vi "ODMR sweep ACCES DAC control low freq.vi"(8 "Save?":bool, 9 "file path (dialog if empty)":path=path "C:/Users/Ouyang Group/Documents/Data/8-12-16/MNP 2 new on CPW 2mW scan 2 x35 y103 ODMR B0.5V T90 rf", 10 "Cluster":T1={"Freq start"=50000000.0, "Freq End"=1000000000.0, "Freq Step"=5000000.0, "Power (dbm)"=-4.0, "number of samples per channel"=200}, 11 "Dot Tracking Cluster":T3={"RS232 settings"={"Portnumber"=12, "Baudrate"=5}, "X Parameters"={"Number of X Steps"=200, "Max X (V)"=2.0, "Min X (V)"=-2.0}, "Y Parameters"={"Number of Y Steps"=200, "Max Y (V)"=2.0, "Min Y (V)"=-2.0}, "X Pos"=75.0, "Y Pos"=145.0, "Z Pos"=52.78, "Tracking interval"=150.0} {"RS232 settings"."Portnumber" items=["COM1", "COM2", "COM3", "COM4", "COM5", "COM6", "COM7", "COM8", "COM9", "COM10", "COM11", "COM12", "COM13", "COM14", "COM15", "COM16", "COM17", "COM18", "COM19", "COM20", "COM21", "COM22", "COM23", "COM24", "COM25", "COM26", "COM27", "COM28", "COM29", "COM30"]; "RS232 settings"."Baudrate" items=["9600", "14400", "19200", "38400", "57600", "115200"]}) -> (0 "Z Position":dbl=31.0, 1 "Y Position":dbl=62.0, 2 "X Position":dbl=97.0, 3 "XY Graph":cluster{"Y":dbl[], "Y":dbl[]}[](graph), 4 "appended array":ext[][](array[numeric]))   [LabVIEW 2012]
uses:
  <vilib>/DAQmx/read.llb/DAQmx Read (Counter 1D DBL 1Chan NSamp).vi
  <vilib>/DAQmx/create/channels.llb/DAQmx Create Channel (CI-Count Edges).vi
  <vilib>/DAQmx/configure/timing.llb/DAQmx Timing (Sample Clock).vi
  <vilib>/Instr/_visa.llb/VISA Configure Serial Port (Instr).vi
  <vilib>/DAQmx/miscellaneous.llb/DAQmx Fill In Error Info.vi
  <vilib>/Utility/file.llb/Write To Spreadsheet File (DBL).vi
  <resource>/objmgr/daqmx.rc
panel:
  in  "Serial Cluster":T2={"baud rate"=4800, "VISA resource name"="COM8", "data bits"=8, "parity"=0, "stop bits"=10, "flow control"=0} {"flow control" items=["None"=0, "XON/XOFF"=1, "RTS/CTS"=2, "DTR/DSR"=4]; "stop bits" items=["1.0"=10, "1.5"=15, "2.0"=20]; "parity" items=["None", "Odd", "Even", "Mark", "Space"]; "data bits" min=5 max=8 step=1}
  in  "stop":bool
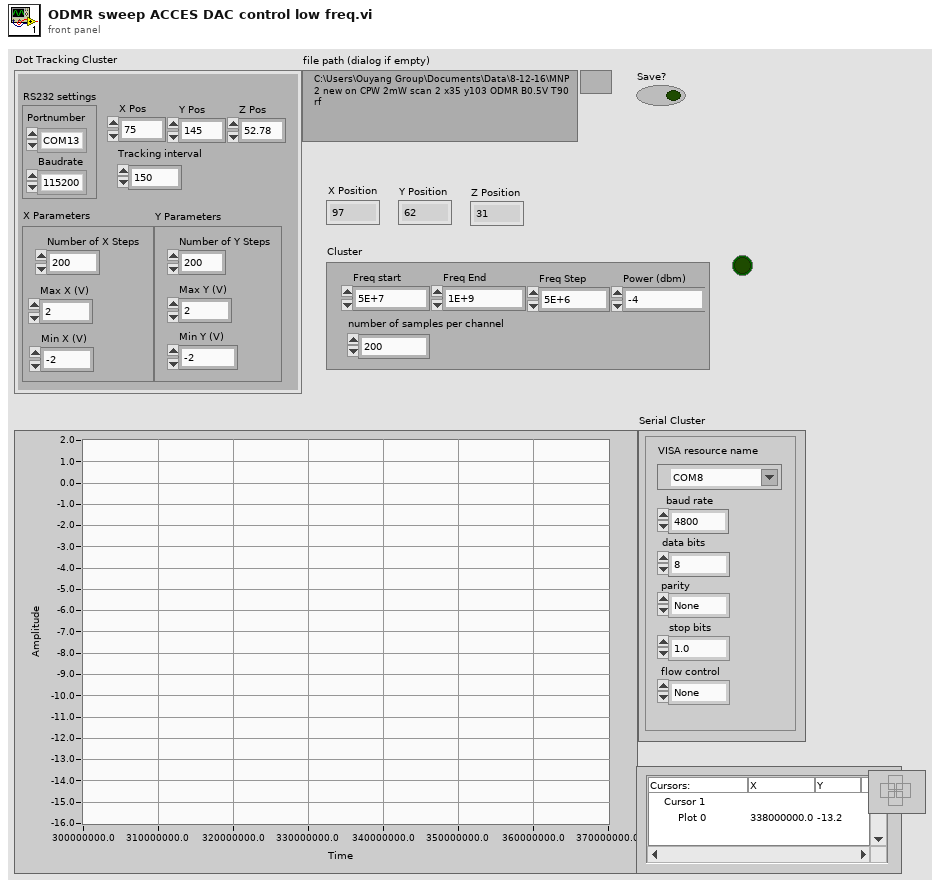
[diagram p1: front panel]
types:
  T1 = cluster{"Freq start":dbl, "Freq End":dbl, "Freq Step":dbl, "Power (dbm)":dbl, "number of samples per channel":i32}
  T2 = cluster{"baud rate":u32, "VISA resource name":refnum<visa-resource-name>, "data bits":u16, "parity":u16, "stop bits":u16, "flow control":u16}
  T3 = cluster{"RS232 settings":cluster{"Portnumber":i32, "Baudrate":u16}, "X Parameters":cluster{"Number of X Steps":i32, "Max X (V)":dbl, "Min X (V)":dbl}, "Y Parameters":cluster{"Number of Y Steps":i32, "Max Y (V)":dbl, "Min Y (V)":dbl}, "X Pos":dbl, "Y Pos":dbl, "Z Pos":dbl, "Tracking interval":dbl}
  T4 = cluster{"Number of X Steps":i32, "Max X (V)":dbl, "Min X (V)":dbl}
  T5 = cluster{"Number of Y Steps":i32, "Max Y (V)":dbl, "Min Y (V)":dbl}
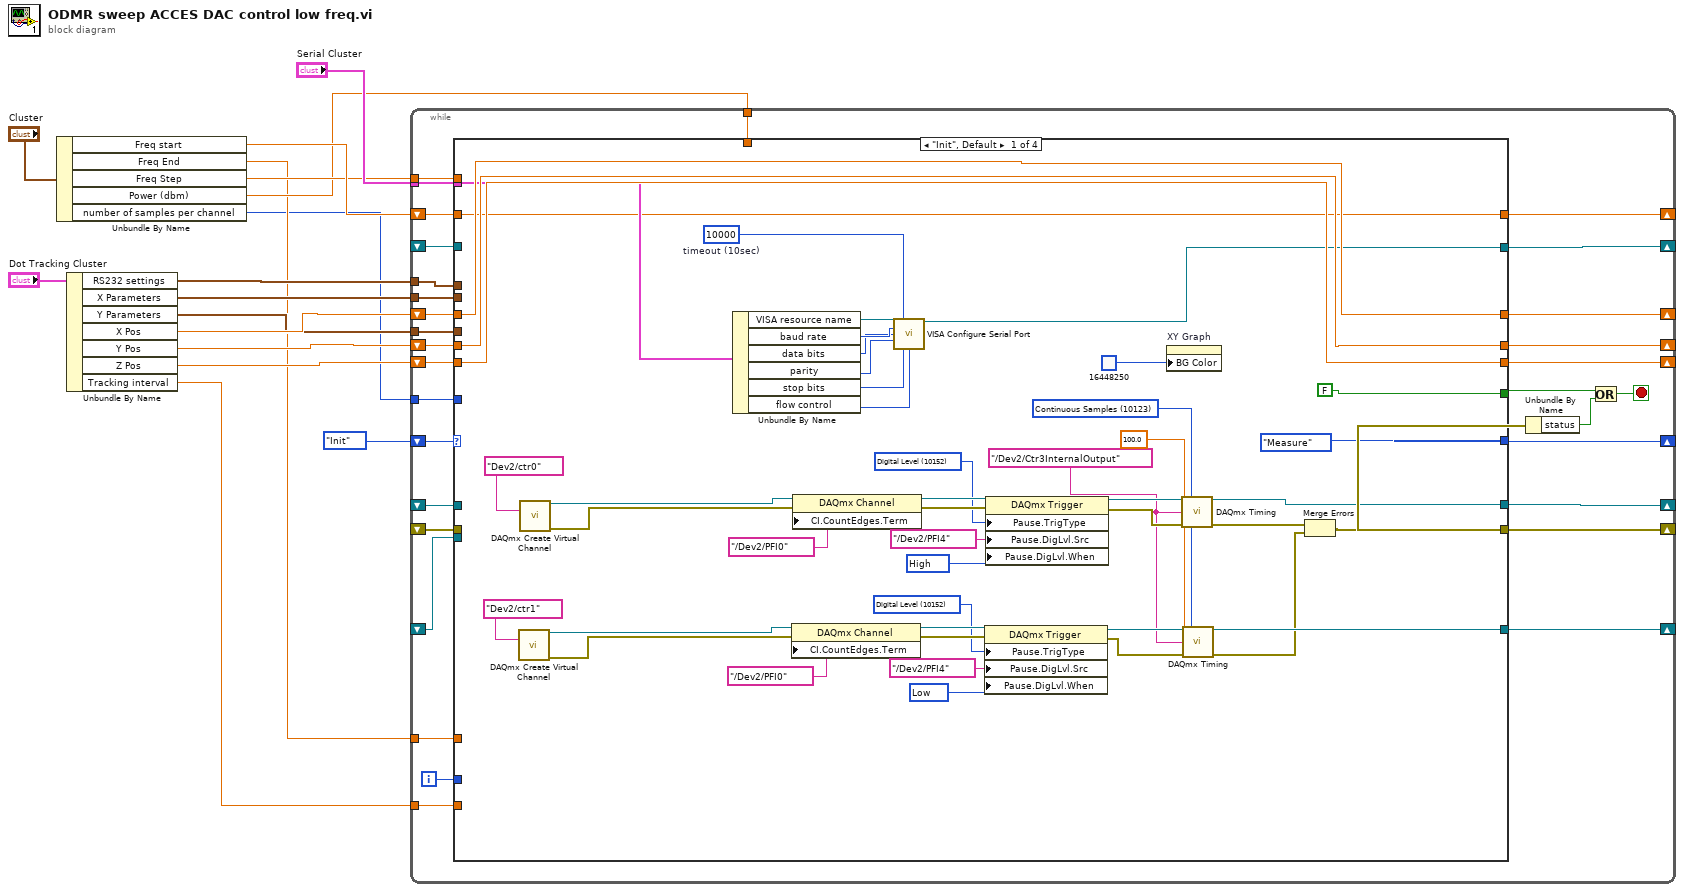
[diagram p0: block diagram]
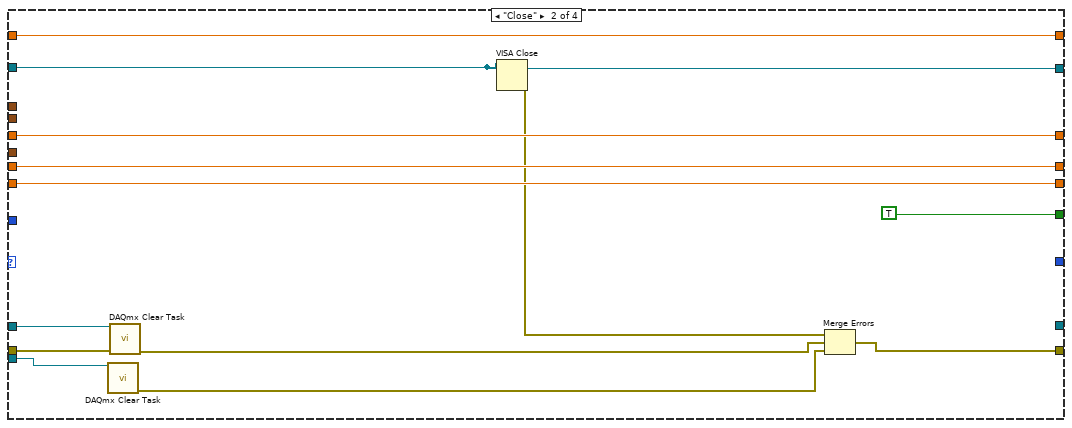
[diagram p2: hidden frame]
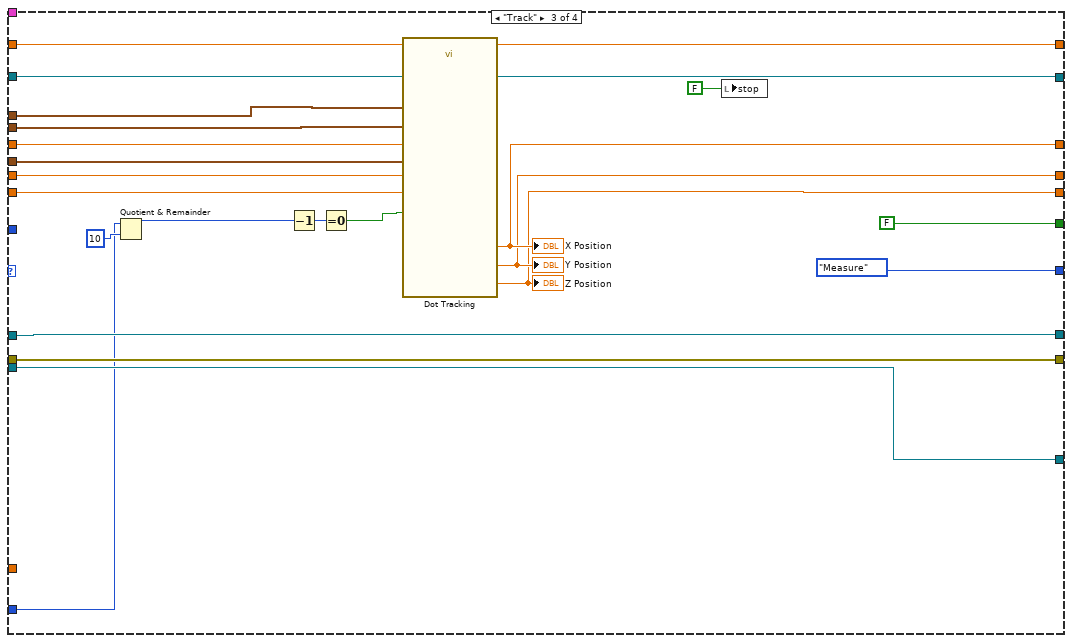
[diagram p3: hidden frame]
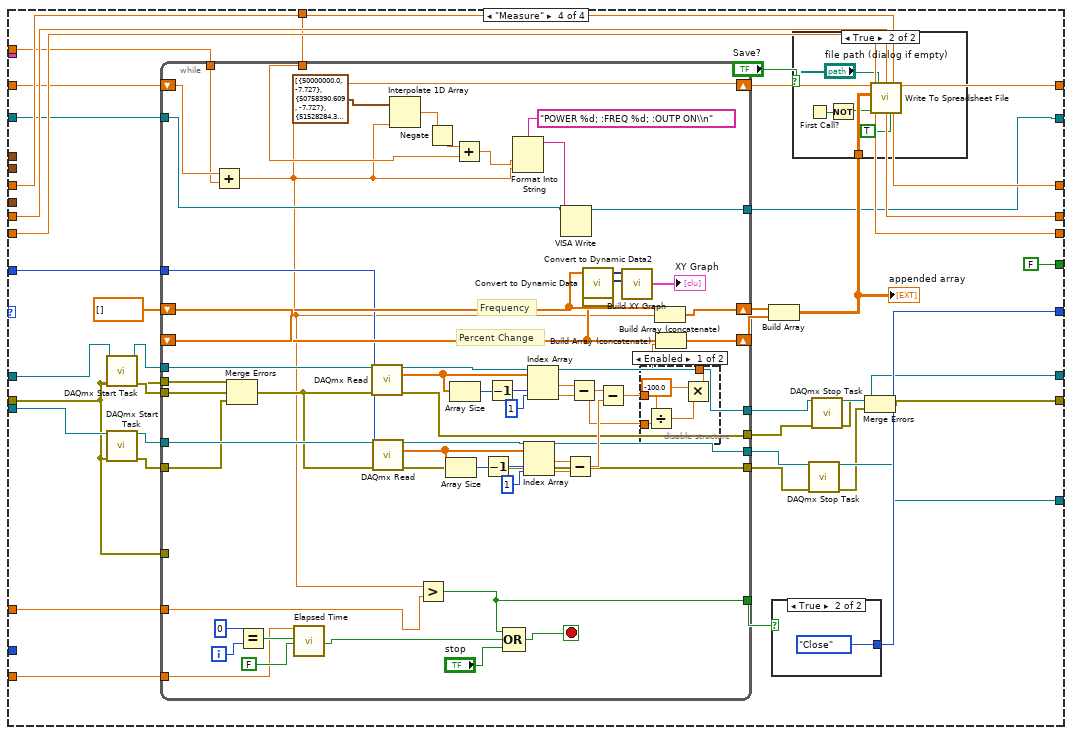
[diagram p4: hidden frame]
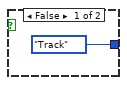
[diagram p6: hidden frame]
diagram:
  n1 = Unbundle By Name("Cluster") -> ("Freq start"=w5:dbl, "Freq End"=w2:dbl, "Freq Step"=w4:dbl, "Power (dbm)"=w3:dbl, "number of samples per channel"=w1:i32)
  n2 = Unbundle By Name("Dot Tracking Cluster") -> ("RS232 settings"=w11:cluster{"Portnumber":i32, "Baudrate":u16}, "X Parameters"=w10:T4, "Y Parameters"=w9:T5, "X Pos"=w14:dbl, "Y Pos"=w13:dbl, "Z Pos"=w12:dbl, "Tracking interval"=w8:dbl)
  n3 = while {
    shift-right: [w44] -> _
    shift-left: enum16{"Init", "Measure", "Track", "Close"}."Init" -> [w47]
    shift-right: [w46] -> _
    shift-left: _ -> [w43]
    shift-right: [w45] -> _
    shift-left: _ -> [w42]
    shift-right: [w40] -> _
    shift-left: _ -> [w41]
    shift-right: [w33] -> _
    shift-left: w14 -> [w36]
    shift-right: [w32] -> _
    shift-left: w13 -> [w35]
    shift-right: [w31] -> _
    shift-left: w12 -> [w34]
    tunnel: w11 -> [w30]
    tunnel: w10 -> [w29]
    tunnel: w9 -> [w28]
    tunnel: w8 -> [w27]
    tunnel: "Serial Cluster" -> [w26]
    tunnel: w3 -> [w25]
    shift-right: [w21] -> _
    shift-left: w5 -> [w24]
    shift-right: [w23] -> _
    shift-left: _ -> [w22]
    tunnel: w4 -> [w20]
    tunnel: w2 -> [w19]
    tunnel: w1 -> [w18]
    i -> [w17]
    stop <- w39 stop-if-true
    n4 = case shown="\"Init\", Default" w47 {
      tunnel: [FALSE TRUE FALSE FALSE] -> w38
      tunnel: [w69 _ w128 w154] -> w46
      tunnel: [w68 _ w127 w151] -> w45
      tunnel: [w65 w101 w122 w164] -> w40
      tunnel: [enum16{"Init", "Measure", "Track", "Close"}."Measure" _ enum16{"Init", "Measure", "Track", "Close"}."Measure" w163] -> w44
      tunnel: w43 -> [_ w105 w128 w160]
      tunnel: w42 -> [_ w103 w127 w157]
      tunnel: w41 -> [_ w104 w122 w141]
      tunnel: w36 -> [w61 w99 w118 w146]
      tunnel: w35 -> [w60 w98 w117 w145]
      tunnel: w34 -> [w59 w97 w116 w144]
      tunnel: [w61 w99 w115 w146] -> w33
      tunnel: [w60 w98 w114 w145] -> w32
      tunnel: [w59 w97 w113 w144] -> w31
      tunnel: w30 -> [_ _ w112 _]
      tunnel: w29 -> [_ _ w111 _]
      tunnel: w28 -> [_ _ w110 _]
      tunnel: w27 -> [_ _ _ w140]
      tunnel: w26 -> [w51 _ _ _]
      tunnel: w25 -> [_ _ _ w136]
      tunnel: w24 -> [w49 w94 w108 w135]
      tunnel: [w50 w95 w109 w133] -> w23
      tunnel: w22 -> [_ w95 w109 w134]
      tunnel: [w49 w94 w108 w132] -> w21
      tunnel: w20 -> [_ _ _ w131]
      tunnel: w19 -> [_ _ _ w130]
      tunnel: w18 -> [_ _ _ w129]
      tunnel: w17 -> [_ _ w107 _]
      frame "Init", Default {
        w48 = 100.0 ("rate")
        w58 = u32 10000  # timeout (10sec)
        w70 = tag "/Dev2/Ctr3InternalOutput" ("source")
        w71 = 10123 items=["Finite Samples"=10178, "Continuous Samples"=10123, "Hardware Timed Single Point"=12522] ("sample mode")
        w76 = 10214 items=["High"=10192, "Low"=10214] ("Pause.DigLvl.When")
        w78 = 10152 items=["Analog Level"=10101, "Analog Window"=10103, "Digital Level"=10152, "Digital Pattern"=10398, "None"=10230] ("Pause.TrigType")
        w85 = 10192 items=["High"=10192, "Low"=10214] ("Pause.DigLvl.When")
        w87 = 10152 items=["Analog Level"=10101, "Analog Window"=10103, "Digital Level"=10152, "Digital Pattern"=10398, "None"=10230] ("Pause.TrigType")
        n5 = call-poly <vilib>:"DAQmx Create Virtual Channel.vi"("counter"=tag "Dev2/ctr1") -> ("task out"=w83:refnum<k21>, "error out"=w82:errorcluster)  [unwired: 13 in]
        n6 = call-poly <vilib>:"DAQmx Create Virtual Channel.vi"("counter"=tag "Dev2/ctr0") -> ("task out"=w92:refnum<k21>, "error out"=w91:errorcluster)  [unwired: 13 in]
        n7 = Unbundle By Name(w51) -> ("VISA resource name"=w57:refnum<visa-resource-name>, "baud rate"=w56:u32, "data bits"=w55:u16, "parity"=w54:u16, "stop bits"=w53:u16, "flow control"=w52:u16)
        n8 = property class="DAQmx Channel"(reference=w83, error in=w82, "CI.CountEdges.Term"=tag "/Dev2/PFI0") -> (reference out=w80:refnum<k21>, error out=w79:errorcluster)
        n9 = property class="DAQmx Channel"(reference=w92, error in=w91, "CI.CountEdges.Term"=tag "/Dev2/PFI0") -> (reference out=w89:refnum<k21>, error out=w88:errorcluster)
        n10 = call-poly "VISA Configure Serial Port"("VISA resource name"=w57, "timeout (10sec)"=w58, "baud rate (9600)"=w56, "data bits (8)"=w55, "parity (0:none)"=w54, "stop bits (10: 1 bit)"=w53, "flow control (0:none)"=w52) -> ("VISA resource name out"=w50:refnum<visa-resource-name>)  [unwired: 2 in, 6 out]
        n11 = property class="DAQmx Trigger"(reference=w80, error in=w79, "Pause.TrigType"=w78, "Pause.DigLvl.Src"=tag "/Dev2/PFI4", "Pause.DigLvl.When"=w76) -> (reference out=w73:refnum<k21>, error out=w72:errorcluster)
        n12 = property class="DAQmx Trigger"(reference=w89, error in=w88, "Pause.TrigType"=w87, "Pause.DigLvl.Src"=tag "/Dev2/PFI4", "Pause.DigLvl.When"=w85) -> (reference out=w75:refnum<k21>, error out=w74:errorcluster)
        n13 = property on="XY Graph" class="XYGraph (strict)"("BG Color"=u32 16448250) -> ()  [unwired: 2 in, 2 out]
        n14 = call-poly <vilib>:"DAQmx Timing.vi"("task/channels in"=w75, "sample mode"=w71, "rate"=w48, "source"=w70, "error in"=w74) -> ("task out"=w69:refnum<k21>, "error out"=w67:errorcluster)  [unwired: 9 in]
        n15 = call-poly <vilib>:"DAQmx Timing.vi"("task/channels in"=w73, "sample mode"=w71, "rate"=w48, "source"=w70, "error in"=w72) -> ("task out"=w68:refnum<k21>, "error out"=w66:errorcluster)  [unwired: 9 in]
        n16 = Merge Errors(w67, w66) -> (w65:errorcluster)
      }
      frame "Close" {
        n17 = call <vilib>:"DAQmx Clear Task.vi"("task in"=w103) -> ("error out"=w102:errorcluster)  [unwired: 14 in]
        n18 = call <vilib>:"DAQmx Clear Task.vi"("task in"=w105, "error in"=w104) -> ("error out"=w100:errorcluster)  [unwired: 13 in]
        n19 = VISA Close(VISA resource name=w95) -> (error out=w96:errorcluster)  [unwired: 1 in]
        n20 = Merge Errors(w96, w100, w102) -> (w101:errorcluster)
      }
      frame "Track" {
        n21 = Quotient & Remainder(x=w107, y=10) -> (x-y*floor(x/y)=w125:i32)  [unwired: 1 out]
        n22 = Decrement(x=w125) -> (x-1=w126:i32)
        n23 = Equal To 0?(x=w126) -> (x = 0?=w123:bool)
        n24 = call "Dot Tracking.vi"("X"=w111, "Y Parameters"=w110, "RS232 settings"=w112, "X Pos"=w118, "Y pos"=w117, "Z Pos"=w116, "Z-track?"=w123) -> ("X Position"=w115:dbl, "Y Position"=w114:dbl, "Z Position"=w113:dbl)  [unwired: 2 in, 4 out]
        "X Position" <- w115
        "Y Position" <- w114
        "Z Position" <- w113
        n25 = local write "stop"(FALSE ("stop")) -> ()
      }
      frame "Measure" {
        w147 = dbl[] []
        n26 = call <vilib>:"DAQmx Start Task.vi"("task/channels in"=w160, "error in"=w141) -> ("task out"=w158:refnum<k21>, "error out"=w159:errorcluster)  [unwired: 12 in]
        n27 = call <vilib>:"DAQmx Start Task.vi"("task/channels in"=w157, "error in"=w141) -> ("task out"=w156:refnum<k21>, "error out"=w155:errorcluster)  [unwired: 12 in]
        n28 = while {
          shift-right: [w214] -> w149
          shift-left: w147 -> [w202]
          shift-right: [w213] -> w139
          shift-left: w147 -> [w204]
          tunnel: w156 -> [w210]
          tunnel: [w209] -> w153
          tunnel: [w208] -> w162
          tunnel: [w205] -> w161
          tunnel: w159 -> [w207]
          tunnel: w158 -> [w206]
          tunnel: w155 -> [w191]
          tunnel: w141 -> [w186]
          tunnel: [w189] -> w143
          tunnel: [w188] -> w142
          tunnel: w141 -> [_]
          tunnel: w140 -> [w187]
          tunnel: w136 -> [w174]
          shift-right: [w172] -> w132
          shift-left: w135 -> [w183]
          tunnel: w134 -> [w182]
          tunnel: [w181] -> w133
          tunnel: w131 -> [w180]
          tunnel: w130 -> [w179]
          tunnel: w129 -> [w178]
          i -> [w196]
          stop <- w192 stop-if-true
          # "Percent Change"
          # "Frequency"
          n29 = Add(x=w183, y=w180) -> (x+y=w172:dbl)
          n30 = Merge Errors(w186, w207, w191) -> (w190:errorcluster)
          n31 = Equal?(x=0, y=w196) -> (x = y?=w195:bool)
          n32 = call "Elapsed Time"("Time Target (s)"=w187, "Reset"=w195, "Auto Reset"=FALSE) -> ("Time has Elapsed"=w194:bool)  [unwired: 9 in, 7 out]
          n33 = call-poly <vilib>:"DAQmx Read.vi"("task/channels in"=w206, "number of samples per channel"=w178, "error in"=w190) -> ("task out"=w208:refnum<k21>, "data"=w227:dbl[], "error out"=w209:errorcluster)  [unwired: 10 in]
          n34 = call-poly <vilib>:"DAQmx Read.vi"("task/channels in"=w210, "number of samples per channel"=w178, "error in"=w190) -> ("task out"=w205:refnum<k21>, "data"=w216:dbl[], "error out"=w188:errorcluster)  [unwired: 10 in]
          n35 = Interpolate 1D Array(1:w172, 2:cluster{dbl, dbl}[] [{50000000.0, -7.727}, {50758390.609, -7.727}, {51528284.344, -7.724}, {52309855.683, -7.721}, {53103281.749, -7.719}, {53908742.353, -7.717}, {54726420.031, -7.713}, {55556500.091, -7.707}, {56399170.65, -7.705}, {57254622.678, -7.704}, {58123050.041, -7.702}, {59004649.547, -7.697}, {59899620.989, -7.692}, {60808167.19, -7.69}, {61730494.048, -7.69}, {62666810.588, -7.693}, {63617329.0, -7.696}, {64582264.698, -7.699}, {65561836.359, -7.703}, {66556265.979, -7.704}, {67565778.921, -7.705}, {68590603.965, -7.708}, {69630973.363, -7.709}, {70687122.889, -7.712}, {71759291.892, -7.711}, {72847723.354, -7.714}, {73952663.939, -7.719}, {75074364.056, -7.721}, {76213077.909, -7.722}, {77369063.56, -7.719}, {78542582.985, -7.72}, {79733902.131, -7.722}, {80943290.983, -7.723}, {82171023.618, -7.722}, {83417378.271, -7.722}, {84682637.396, -7.723}, {85967087.735, -7.722}, {87271020.376, -7.72}, {88594730.821, -7.72}, {89938519.058, -7.719}, {91302689.623, -7.721}, {92687551.67, -7.719}, {94093419.045, -7.716}, {95520610.353, -7.713}, {96969449.03, -7.712}, {98440263.419, -7.712}, {99933386.846, -7.713}, {101449157.688, -7.711}, {102987919.457, -7.711}, {104550020.876, -7.71}, {106135815.956, -7.714}, {107745664.078, -7.718}, {109379930.073, -7.723}, {111038984.309, -7.729}, {112723202.767, -7.734}, {114432967.135, -7.742}, {116168664.887, -7.752}, {117930689.377, -7.764}, {119719439.924, -7.778}, {121535321.903, -7.791}, {123378746.838, -7.806}, {125250132.497, -7.818}, {127149902.982, -7.832}, {129078488.829, -7.846}, {131036327.104, -7.86}, {133023861.502, -7.875}, {135041542.448, -7.885}, {137089827.2, -7.896}, {139169179.951, -7.905}, {141280071.933, -7.915}, {143422981.529, -7.923}, {145598394.374, -7.933}, {147806803.474, -7.942}, {150048709.307, -7.951}, {152324619.948, -7.961}, {154635051.173, -7.966}, {156980526.585, -7.971}, {159361577.728, -7.974}, {161778744.208, -7.98}, {164232573.814, -7.986}, {166723622.647, -7.99}, {169252455.241, -7.993}, {171819644.693, -7.997}, {174425772.792, -8.008}, {177071430.153, -8.015}, {179757216.347, -8.027}, {182483740.043, -8.031}, {185251619.137, -8.042}, {188061480.902, -8.045}, {190913962.122, -8.052}, {193809709.242, -8.067}, {196749378.51, -8.095}, {199733636.129, -8.136}, {202763158.407, -8.183}, {205838631.911, -8.231}, {208960753.619, -8.277}, {212130231.082, -8.319}, {215347782.584, -8.359}, {218614137.303, -8.406}, {221930035.478, -8.46}, {225296228.572, -8.517}, {228713479.452, -8.567}, {232182562.551, -8.604}, {235704264.05, -8.632}, {239279382.057, -8.653}, {242908726.782, -8.683}, {246593120.726, -8.713}, {250333398.866, -8.731}, {254130408.842, -8.746}, {257985011.152, -8.765}, {261898079.346, -8.804}, {265870500.223, -8.841}, {269903174.034, -8.865}, {273997014.684, -8.879}, {278152949.94, -8.888}, {282371921.641, -8.905}, {286654885.913, -8.935}, {291002813.382, -8.96}, {295416689.399, -8.977}, {299897514.258, -8.973}, {304446303.427, -8.971}, {309064087.776, -8.976}, {313751913.81, -8.988}, {318510843.909, -8.988}, {323341956.566, -8.971}, {328246346.633, -8.947}, {333225125.566, -8.921}, {338279421.684, -8.909}, {343410380.416, -8.918}, {348619164.566, -8.95}, {353906954.576, -8.982}, {359274948.791, -9.004}, {364724363.734, -9.02}, {370256434.38, -9.037}, {375872414.435, -9.048}, {381573576.62, -9.043}, {387361212.962, -9.037}, {393236635.085, -9.028}, {399201174.508, -9.018}, {405256182.944, -8.977}, {411403032.611, -8.91}, {417643116.539, -8.825}, {423977848.888, -8.754}, {430408665.267, -8.707}, {436937023.062, -8.718}, {443564401.761, -8.787}, {450292303.296, -8.88}, {457122252.377, -8.969}, {464055796.844, -9.032}, {471094508.01, -9.084}, {478239981.026, -9.11}, {485493835.234, -9.134}, {492857714.54, -9.169}, {500333287.785, -9.199}, {507922249.121, -9.245}, {515626318.396, -9.313}, {523447241.548, -9.435}, {531386790.992, -9.56}, {539446766.032, -9.655}, {547628993.259, -9.685}, {555935326.972, -9.668}, {564367649.595, -9.637}, {572927872.103, -9.632}, {581617934.459, -9.69}, {590439806.048, -9.817}, {599395486.128, -9.996}, {608487004.282, -10.149}, {617716420.876, -10.193}, {627085827.527, -10.1}, {636597347.578, -9.915}, {646253136.579, -9.736}, {656055382.774, -9.647}, {666006307.599, -9.672}, {676108166.182, -9.754}, {686363247.858, -9.807}, {696773876.687, -9.778}, {707342411.98, -9.688}, {718071248.83, -9.611}, {728962818.663, -9.595}, {740019589.781, -9.667}, {751244067.926, -9.777}, {762638796.849, -9.854}, {774206358.879, -9.862}, {785949375.517, -9.817}, {797870508.026, -9.804}, {809972458.034, -9.882}, {822257968.147, -10.045}, {834729822.57, -10.214}, {847390847.738, -10.287}, {860243912.958, -10.298}, {873291931.057, -10.345}, {886537859.043, -10.509}, {899984698.778, -10.574}, {913635497.652, -10.699}, {927493349.279, -10.743}, {941561394.198, -10.672}, {955842820.579, -10.575}, {970340864.953, -10.477}, {985058812.941, -10.388}, {1000000000.0, -10.309}] ("Array")) -> (0:w176:dbl)
          n36 = Greater?(x=w172, y=w179) -> (0:w189:bool)
          n37 = Negate(x=w176) -> (-x=w175:dbl)
          n38 = Array Size(array=w216) -> (size(s)=w221:i32)
          n39 = Array Size(array=w227) -> (size(s)=w226:i32)
          n40 = Add(x=w175, y=w174) -> (x+y=w173:dbl)
          n41 = Decrement(x=w221) -> (x-1=w220:i32)
          n42 = Decrement(x=w226) -> (x-1=w225:i32)
          n43 = Compound Arithmetic op=OR(w189, w194, "stop") -> (w192:bool)
          n44 = Format Into String(format string="POWER %d; :FREQ %d; :OUTP ON\\n", w173, w172) -> (resulting string=w184:string)  [unwired: 2 in, 1 out]
          n45 = Index Array(array=w216, index #1=w220, index #2=1 ("index")) -> (element #1=w217:dbl, element #2=w218:dbl)
          n46 = Index Array(array=w227, index #1=w225, index #2=1 ("index")) -> (element #1=w222:dbl, element #2=w223:dbl)
          n47 = VISA Write(VISA resource name=w182, write buffer=w184) -> (VISA resource name out=w181:refnum<visa-resource-name>)  [unwired: 1 in, 2 out]
          n48 = Subtract(x=w217, y=w218) -> (x-y=w215:dbl)
          n49 = Subtract(x=w222, y=w223) -> (x-y=w211:dbl)
          n50 = call "Convert to Dynamic Data"("Array"=w204) -> ("Dynamic Data Type"=w203:dynamicdata)  [unwired: 3 in]
          n51 = call "Convert to Dynamic Data2"("Array"=w202) -> ("Dynamic Data Type"=w201:dynamicdata)  [unwired: 3 in]
          n52 = Subtract(x=w211, y=w215) -> (x-y=w212:dbl)
          n53 = call "Build XY Graph"("Y Input"=w201, "X Input"=w203) -> ("XY Graph"=→"XY Graph":cluster{"Y":dbl[], "Y":dbl[]}[])  [unwired: 3 in, 6 out]
          n54 = disable-structure shown="Enabled" {
            disable-tunnel: w212 -> [w232 w233]
            disable-tunnel: w211 -> [w231 _]
            disable-tunnel: [w229 w233] -> w199
            frame Enabled {
              n55 = Divide(x=w232, y=w231) -> (x/y=w230:dbl)
              n56 = Multiply(x=-100.0, y=w230) -> (x*y=w229:dbl)
            }
            frame Disabled {
            }
          }
          n57 = Build Array (concatenate)(w204, w172) -> (w213:dbl[])
          n58 = Build Array (concatenate)(w202, w199) -> (w214:dbl[])
        }
        n59 = Build Array(w139, w149) -> (w148:dbl[][])
        "appended array" <- w148
        n60 = case shown="True" w143 {
          tunnel: [enum16{"Init", "Measure", "Track", "Close"}."Track" enum16{"Init", "Measure", "Track", "Close"}."Close"] -> w163
          frame False {
          }
          frame True {
          }
        }
        n61 = case shown="True" "Save?" {
          tunnel: w148 -> [_ w169]
          frame False {
          }
          frame True {
            n62 = First Call?() -> (First Call?: T/F=w168:bool)
            n63 = Not(x=w168) -> (.not. x?=w167:bool)
            n64 = call-poly <vilib>:"Write To Spreadsheet File.vi"("transpose? (no:F)"=TRUE, "append to file? (new file:F)"=w167, "2D data"=w169, "file path (dialog if empty)"="file path (dialog if empty)") -> ()  [unwired: 4 in, 1 out]
          }
        }
        n65 = call <vilib>:"DAQmx Stop Task.vi"("task/channels in"=w161, "error in"=w142) -> ("task out"=w151:refnum<k21>, "error out"=w150:errorcluster)  [unwired: 12 in]
        n66 = call <vilib>:"DAQmx Stop Task.vi"("task/channels in"=w162, "error in"=w153) -> ("task out"=w154:refnum<k21>, "error out"=w152:errorcluster)  [unwired: 12 in]
        n67 = Merge Errors(w152, w150) -> (w164:errorcluster)
      }
    }
    n68 = Unbundle By Name(w40) -> ("status"=w37:bool)
    n69 = Or(x=w38, y=w37) -> (x .or. y?=w39:bool)
  }
